vi "FSM_main_v2.vi"() -> ()   [LabVIEW 2016]
uses:
  Microgrid project/labview/Untitled Project 3/controls/Functional Global Operation.ctl
  Microgrid project/labview/Untitled Project 3/support/Message Queue/Message Queue.lvlib
panel:
  out "Bool of state":bool[](array[boolean])
  in  "Event manual panel":bool
  in  "Manual turn off":bool
  out "Current Time":string
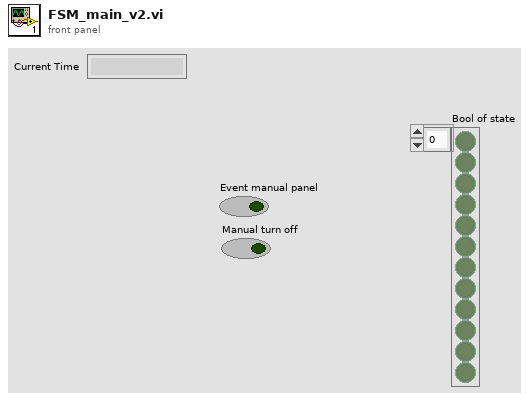
[diagram p1: front panel]
types:
  T1 = typedef "Functional Global Operation.ctl" = enum16{"Initialize", "Read", "Write"}
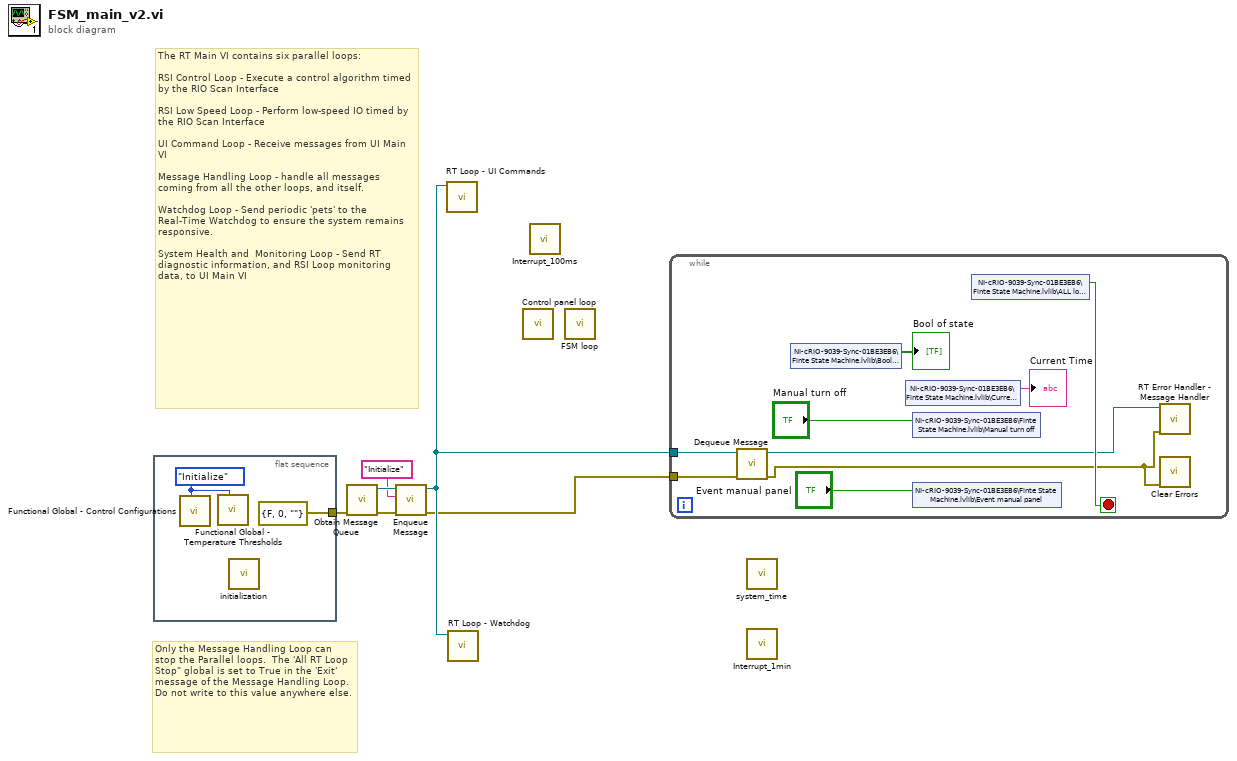
[diagram p0: block diagram]
diagram:
  # "The RT Main VI contains six parallel loops:\n\nRSI Control Loop - Execute a control algorithm timed by the RIO Scan Interface\n\nRSI Low Speed Loop - Perform low-speed IO timed by the RIO Scan Interface\n\nUI Command Loop - Receive messages from UI Main VI\n\nMessage Handling Loop - handle all messages coming from all the other loops, and itself.\n\nWatchdog Loop - Send periodic 'pets' to the Real-Time Watchdog to ensure the system remains responsive.\n\nSystem Health and  Monitoring Loop - Send RT diagnostic information, and RSI Loop monitoring data, to UI Main VI"
  # "Only the Message Handling Loop can stop the Parallel loops.  The 'All RT Loop Stop\" global is set to True in the 'Exit' message of the Message Handling Loop.  Do not write to this value anywhere else."
  n1 = flat-sequence {
    tunnel: [errorcluster {"status"=FALSE, "code"=0, "source"=""} ("error constant")] -> w4
    frame #0 {
      w7 = Functional_Global_Operation."Initialize" ("Functional Global Operation (Read)")
      n2 = call "Functional Global - Control Configurations.vi"("Functional Global Operation (Read)"=w7) -> ()  [unwired: 10 in, 1 out]
      n3 = call "Functional Global - Temperature Thresholds.vi"("Functional Global Operation (Read)"=w7) -> ()  [unwired: 10 in, 1 out]
      n4 = call "initialization.vi"() -> ()  [unwired: 12 in]
    }
  }
  n5 = call "Obtain Message Queue.vi"("error in (no error)"=w4) -> ("error out"=w3:errorcluster, "Message Queue"=w6:refnum<queue>)  [unwired: 9 in]
  n6 = call "Enqueue Message.vi"("error in (no error)"=w3, "Message"="Initialize", "Message Queue"=w6) -> ("error out"=w1:errorcluster, "dup Message Queue"=w2:refnum<queue>)  [unwired: 7 in]
  n7 = call "RT Loop - UI Commands.vi"("Message Queue"=w2) -> ()  [unwired: 11 in]
  n8 = call "RT Loop - Watchdog.vi"("Message Queue"=w2) -> ()  [unwired: 11 in]
  n9 = call "Control panel loop.vi"() -> ()  [unwired: 12 in]
  n10 = call "Interrupt_100ms.vi"() -> ()  [unwired: 11 in, 1 out]
  n11 = call "FSM loop.vi"() -> ()  [unwired: 6 in, 6 out]
  n12 = while {
    tunnel: w2 -> [w12]
    tunnel: w1 -> [w11]
    stop <- w16 stop-if-true
    n13 = call "Dequeue Message.vi"("error in (no error)"=w11, "Message Queue"=w12) -> ("error out"=w9:errorcluster, "dup Message Queue"=w10:refnum<queue>)  [unwired: 6 in, 2 out]
    n14 = shared-variable "NI-cRIO-9039-Sync-01BE3EB6\\Finte State Machine.lvlib\\Bool of state"() -> (→"Bool of state":bool[])  [unwired: 1 in, 1 out]
    n15 = shared-variable "NI-cRIO-9039-Sync-01BE3EB6\\Finte State Machine.lvlib\\Current Time"() -> (→"Current Time":string)  [unwired: 1 in, 1 out]
    n16 = shared-variable "NI-cRIO-9039-Sync-01BE3EB6\\Finte State Machine.lvlib\\Manual turn off"("Manual turn off") -> ()  [unwired: 1 in, 1 out]
    n17 = shared-variable "NI-cRIO-9039-Sync-01BE3EB6\\Finte State Machine.lvlib\\Event manual panel"("Event manual panel") -> ()  [unwired: 1 in, 1 out]
    n18 = shared-variable "NI-cRIO-9039-Sync-01BE3EB6\\Finte State Machine.lvlib\\ALL loop stop"() -> (w16:bool)  [unwired: 1 in, 1 out]
    n19 = call "RT Error Handler - Message Handler.vi"("error in (no error)"=w9, "Message Queue"=w10) -> ()  [unwired: 9 in, 1 out]
    n20 = call <vilib>:"Clear Errors.vi"("error in (no error)"=w9) -> ()  [unwired: 5 in, 2 out]
  }
  n21 = call "system_time.vi"() -> ()  [unwired: 12 in]
  n22 = call "Interrupt_1min.vi"() -> ()  [unwired: 11 in, 1 out]
